vi "LAb7_MSK2.vi"() -> ()   [LabVIEW 2019]
uses:
  <vilib>/addons/Modulation/Digital/General/MT Generate Bits (Galois, PN Order).vi
  <vilib>/addons/Modulation/Analog/support/mod_Set Error Source.vi
  <vilib>/addons/Modulation/Digital/Support/Common/Validators/mod_Generate Bits Validate.vi
  <vilib>/addons/Modulation/Digital/Support/Common/Validators/mod_AWGN Validate.vi
  <vilib>/addons/Modulation/Digital/Impairments/subVIs/mod_createSeeds.vi
  <vilib>/addons/Modulation/Digital/Support/Common/Validators/mod_Validate Samples Per Symbol.vi
  <vilib>/addons/Modulation/Analog/support/Validators/mod_Validate Complex Waveform.vi
  <vilib>/addons/Modulation/Analog/support/Validators/mod_WFErrorHandler.vi
  <vilib>/addons/Modulation/Digital/Support/Common/Validators/mod_Generate Filter Coefficients Validate.vi
  <vilib>/addons/Modulation/Digital/General/subVIs/mod_Generate Filter Coefficients.vi
  <vilib>/addons/Modulation/Digital/General/MT Generate MSK System Parameters.vi
  <vilib>/addons/Modulation/Digital/General/subVIs/mod_Generate Bits PN Sequence.vi
  <vilib>/Analysis/1siggen.llb/Gaussian White Noise (obs 90).vi
  <vilib>/addons/Modulation/Analog/MT Upconvert Baseband (Real).vi
  <vilib>/express/express analysis/Spectral/Block/exnSpectralBlock spectral measurements RMS poly.vi
  <vilib>/express/express analysis/Spectral/Block/exnSpectralBlock spectral measurements RMS DDT.vi
  <vilib>/addons/Modulation/Digital/General/MT Format Eye Diagram (complex).vi
  <vilib>/express/express analysis/Spectral/XNode/ExpressSpectralMeasurementsBlockNode.xnode
  <vilib>/addons/Modulation/niDMT.lvlib
  <vilib>/addons/Modulation/niAMT.lvlib
panel:
  in  "Differential Encoding":u16(ring)=1 items=["disable", "enable"]
  in  "Pulse Shaping Filter":u16(ring) items=["none", "Raised Cosine", "Root Raised Cos", "Gaussian"]
  in  "Tab Control 2":T1(tab)
  out "Baseband Wfm2":cluster{"t0":dbl, "dt":dbl, "Y":dbl[]}(graph)
  out "Baseband Wfm":cluster{"t0":dbl, "dt":dbl, "Y":dbl[]}(graph)
  out "Passband Wfm":waveform(dbl)(graph)
  out "Spectrum(FFT)":dynamicdata(graph)
  in  "Tab Control":enum32{"Constellation", "Eye Diagram"}(tab)
  out "Constellation Graph":T2(graph)
  out "Eye Graph":cluster{"t0":dbl, "dt":dbl, "Y":dbl[]}[](graph)
  in  "carrier frequency (Hz)":dbl min=-0.5 max=0.5 format="%.0p"
  in  "Eb/N0 (dB)":dbl=10.0 format="%.2f"
  in  "stop":bool
  in  "Reset":bool=TRUE
  in  "Symbol Rate(HZ)":dbl=10.0 format="%.0p"
  # "MSK"
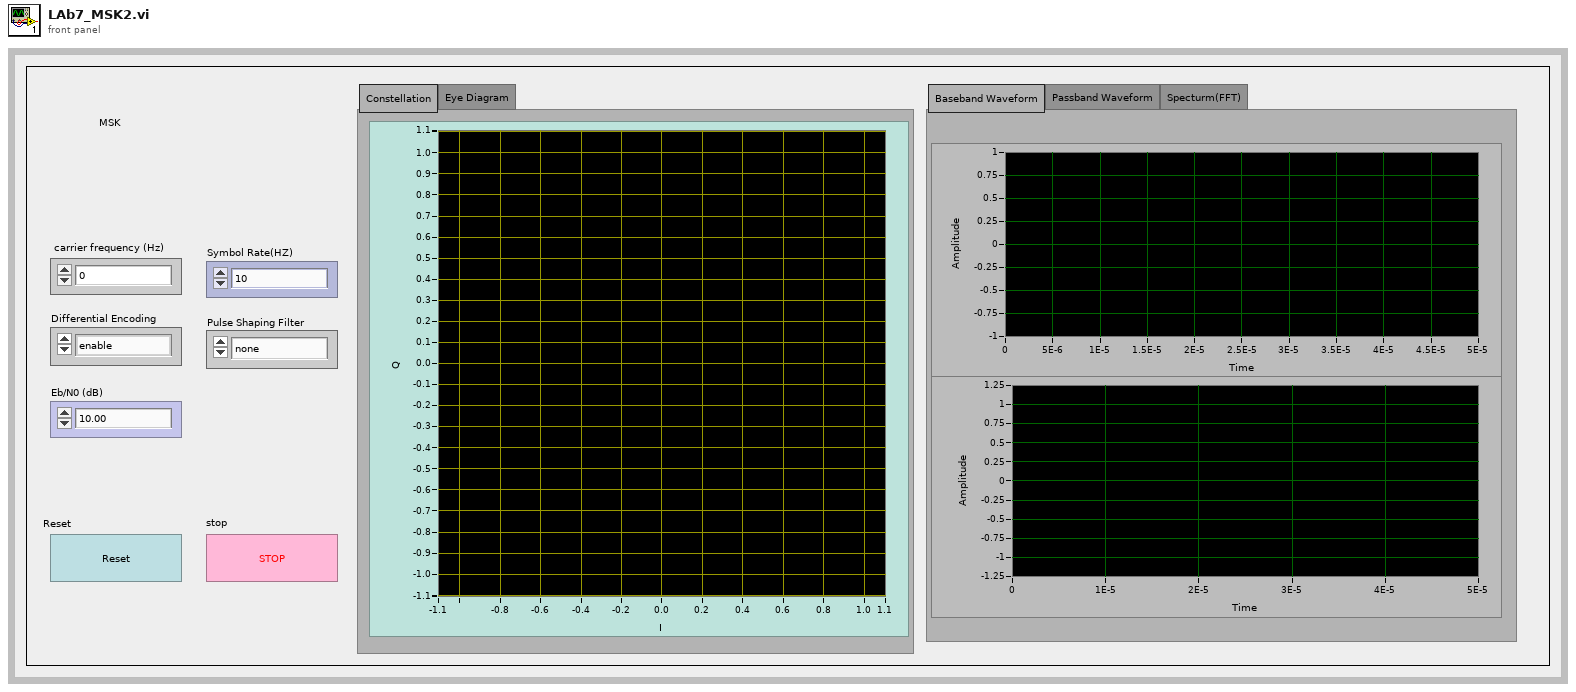
[diagram p1: front panel]
types:
  T1 = enum32{"Baseband Waveform", "Passband Waveform", "Specturm(FFT)"}
  T2 = cluster{"Decimated Array":dbl[], "Decimated Array":dbl[]}[]
  T3 = enum16{"FSK", "PSK", "QAM", "MSK", "PAM", "ASK", "CPM"}
  T4 = cluster{"averaging mode":u16, "weighting mode":u16, "number of averages":u32}
  T5 = cluster{"dB On (F)":bool, "unwrap phase (F)":bool, "convert to degree (F)":bool}
  T6 = cluster{"differential encoding enable":enum16{"disable", "enable"}, "samples per symbol (16)":i32}
  T7 = typedef "niAMT.lvlib/Complex Data Waveform.ctl" = cluster{"t0":dbl, "dt":dbl, "Y":cdb[]}
  T8 = cluster{"constellation":dbl[], "oversampled data":dbl[]}[]
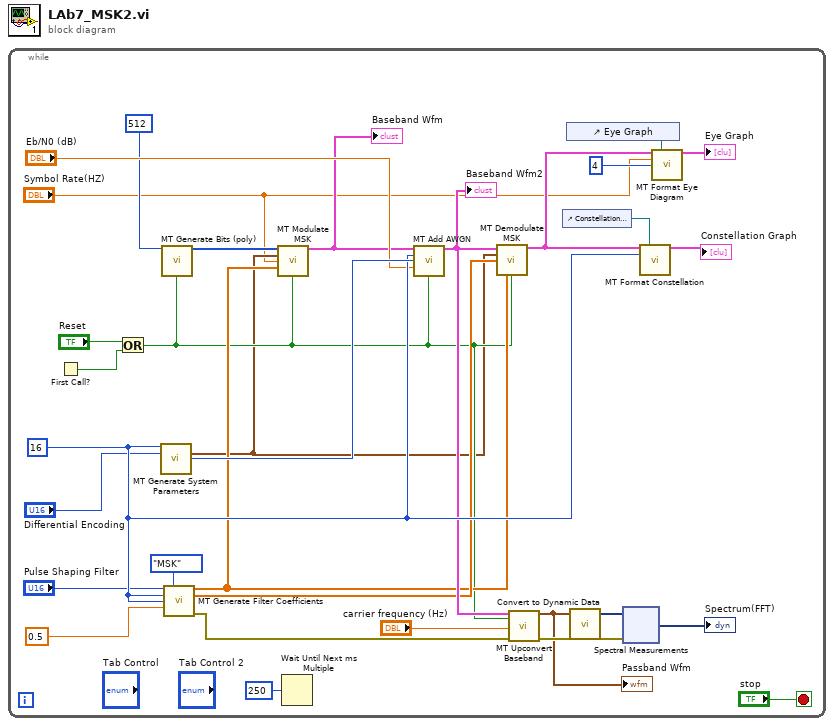
[diagram p0: block diagram]
diagram:
  n1 = while {
    stop <- "stop" stop-if-true
    w18 = 16
    n2 = First Call?() -> (First Call?: T/F=w25:bool)
    n3 = Or(x="Reset", y=w25) -> (x .or. y?=w4:bool)
    n4 = call-poly <vilib>:"MT Generate System Parameters.vi"("samples per symbol (16)"=w18, "differential encoding enable"="Differential Encoding") -> ("MSK system parameters"=w3:T6, "bits per symbol"=w19:i32)  [unwired: 11 in, 1 out]
    n5 = call-poly <vilib>:"MT Generate Bits (poly).vi"("total bits (128)"=512 ("samples per symbol (16)"), "reset? (T)"=w4) -> ("output bit stream"=w20:i8[])  [unwired: 11 in, 2 out]
    n6 = call <vilib>:"MT Generate Filter Coefficients.vi"("pulse shaping filter (none)"="Pulse Shaping Filter", "modulation type"=T3."MSK", "pulse shaping samples per symbol (16)"=w18, "matched samples per symbol (16)"=w18, "filter parameter"=0.5) -> ("pulse shaping filter coefficients"=w5:dbl[], "matched filter coefficients"=w6:dbl[], "error out"=w2:errorcluster)  [unwired: 8 in]
    n7 = call <vilib>:"MT Modulate MSK.vi"("input bit stream"=w20, "MSK system parameters"=w3, "symbol rate (Hz)"="Symbol Rate(HZ)", "pulse shaping filter coefficients"=w5, "reset? (T)"=w4) -> ("output complex waveform"=w12:T7)  [unwired: 8 in, 2 out]
    "Baseband Wfm" <- w12
    n8 = Wait Until Next ms Multiple(millisecond multiple=u32 250) -> ()  [unwired: 1 out]
    n9 = call <vilib>:"MT Add AWGN.vi"("input complex waveform"=w12, "samples per symbol (16)"=w18, "bits per symbol (1)"=w19, "Eb/N0 (10 dB)"="Eb/N0 (dB)", "reset? (T)"=w4) -> ("output complex waveform"=w7:T7)  [unwired: 8 in, 2 out]
    "Baseband Wfm2" <- w7
    n10 = call <vilib>:"MT Demodulate MSK.vi"("input complex waveform"=w7, "MSK system parameters"=w3, "matched filter coefficients"=w6, "pulse shaping filter coefficients"=w5, "reset? (T)"=w4) -> ("recovered complex waveform"=w11:T7)  [unwired: 5 in, 5 out]
    n11 = call-poly <vilib>:"MT Upconvert Baseband.vi"("baseband waveform (complex)"=w7, "reset? (F)"=w4, "carrier frequency (Hz)"="carrier frequency (Hz)", "error in (no error)"=w2) -> ("passband waveform"=w21:waveform(dbl), "error out"=w22:errorcluster)  [unwired: 10 in]
    "Passband Wfm" <- w21
    n12 = control-ref of="Constellation Graph"() -> (w31:refnum<vi>)
    n13 = control-ref of="Eye Graph"() -> (w15:refnum<vi>)
    n14 = call "Convert to Dynamic Data"("Waveform"=w21) -> ("Dynamic Data Type"=w26:dynamicdata)  [unwired: 3 in]
    n15 = xnode "Spectral Measurements"("Signals"=w26, "error in (no error)"=w22) -> ("FFT - (RMS)"=→"Spectrum(FFT)":dynamicdata)  [unwired: 2 out]
    n16 = call <vilib>:"MT Format Constellation.vi"("waveform"=w11, "constellation reference"=w31, "samples per symbol"=w18) -> ("constellation graph"=→"Constellation Graph":T8)  [unwired: 2 in, 10 out]
    n17 = call-poly <vilib>:"MT Format Eye Diagram.vi"("waveform"=w11, "eye diagram reference"=w15, "symbol rate (Hz)"="Symbol Rate(HZ)", "eye length"=4) -> ("eye diagram"=→"Eye Graph":cluster{"t0":dbl, "dt":dbl, "Y":dbl[]}[])  [unwired: 3 in, 8 out]
  }
